vi "stim config to csv (top level vi).vi"() -> ()   [LabVIEW 2021]
uses:
  type-defs/stimulation configuration array (type def).ctl
  type-defs/stimulator configuration line cluster (type def).ctl
  type-defs/port-odor with color cluster (type def).ctl
  type-defs/port-odor ring (type def).ctl
  type-defs/odor color (type def).ctl
  type-defs/odor and manifold config cluster (type def).ctl
  type-defs/manifold configuration cluster array (type def).ctl
  type-defs/manifold configuration cluster (type def).ctl
  type-defs/manifold selection.ctl
  type-defs/single port single odor cluster.ctl
  type-defs/port number (type def).ctl
  type-defs/odor selection (type def).ctl
  type-defs/odor description array (type def).ctl
  type-defs/odor info cluster (type def).ctl
panel:
  out "csv lines out":string[](array[string])
  in  "utilized odor manifold config (none)":T1
  in  "interactive? (T)":bool=TRUE
  out "error out":errorcluster
  in  "error in (no error)":errorcluster
  in  "stim. config array in (none)":T11 {"right odor"."port-odor ring" items=["off"]; "middle odor"."port-odor ring" items=["off"]; "left odor"."port-odor ring" items=["off"]}
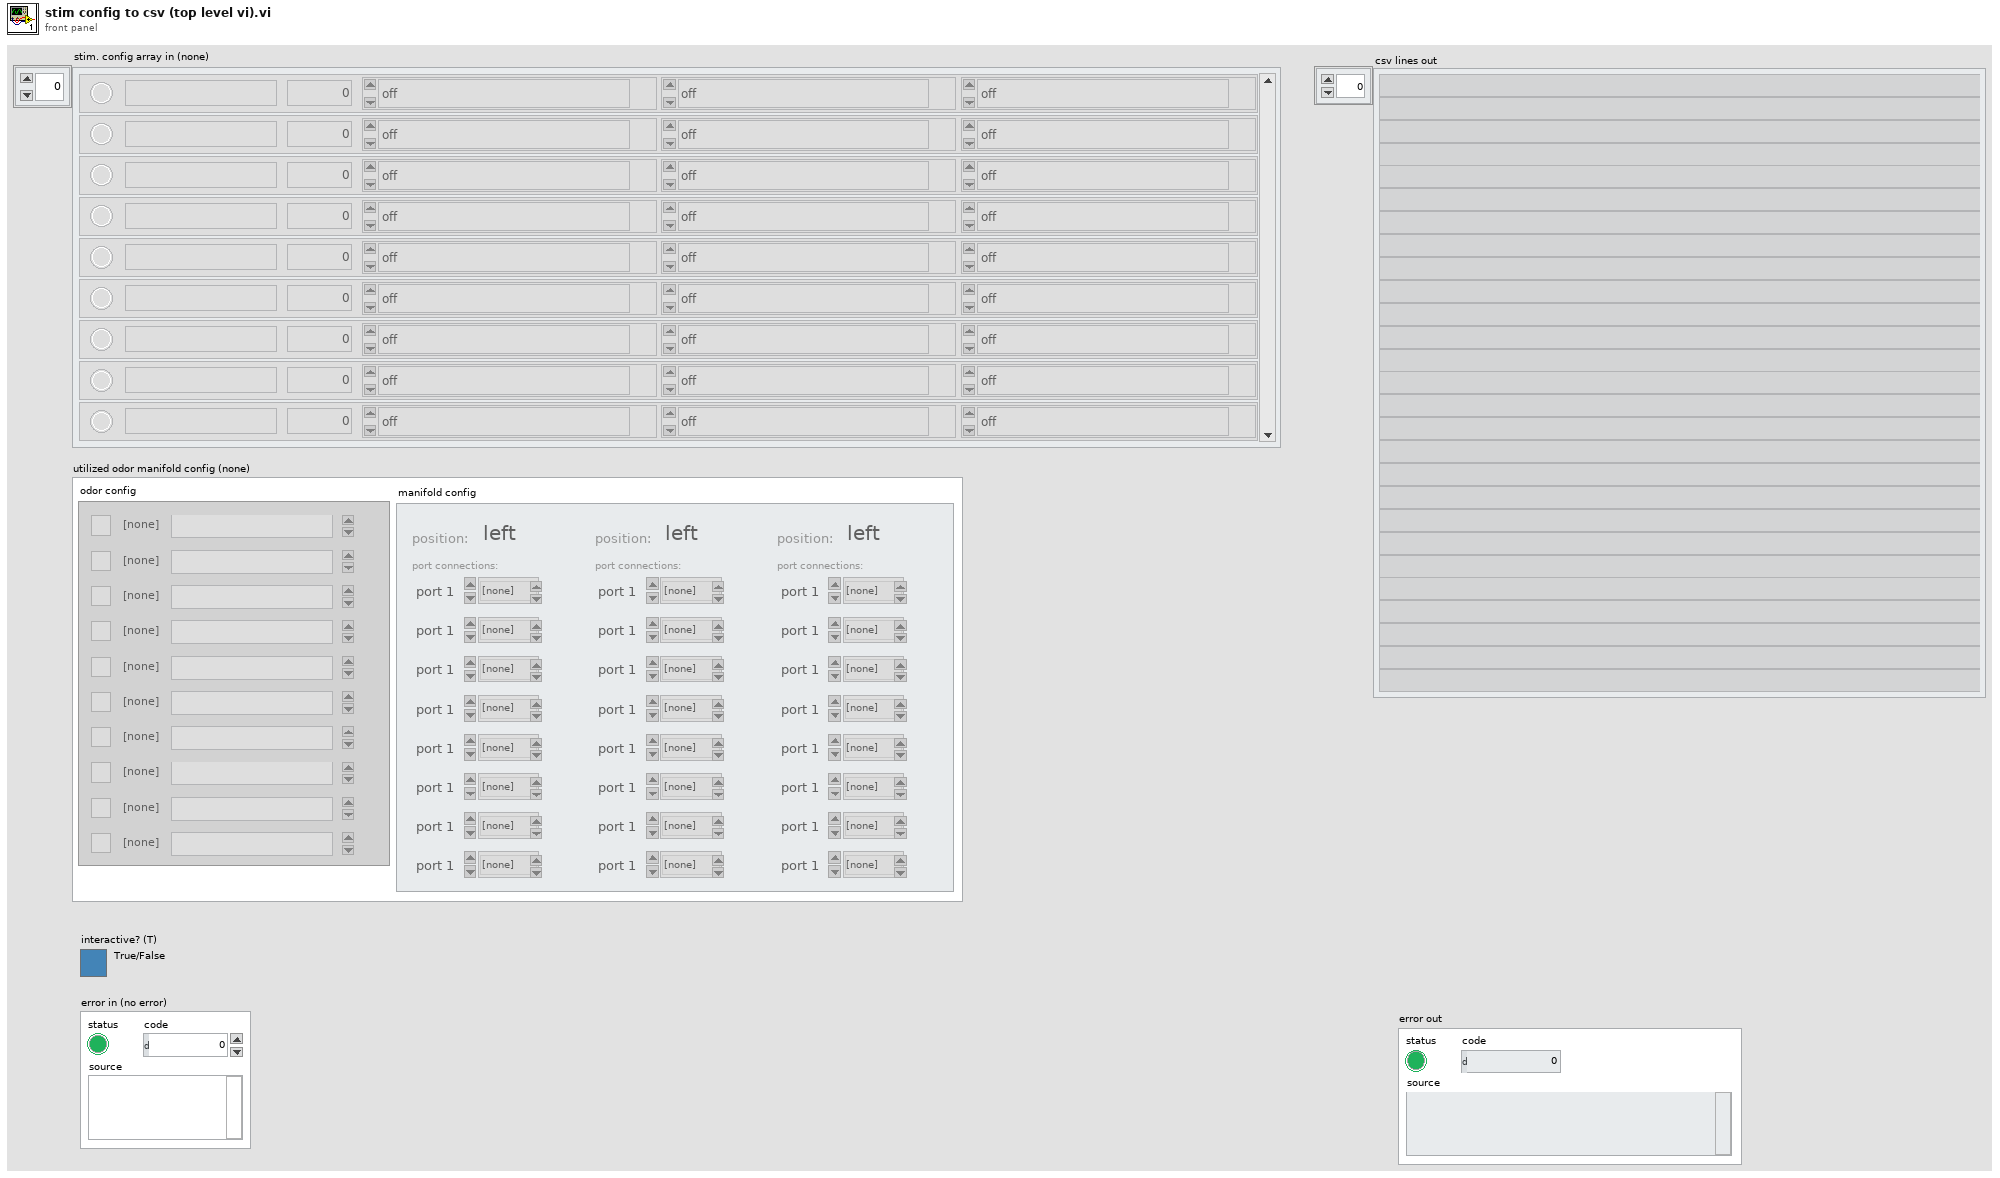
[diagram p1: front panel]
types:
  T1 = typedef "odor and manifold config cluster (type def).ctl" = cluster{"manifold config":T2, "odor config":T9}
  T2 = typedef "manifold configuration cluster array (type def).ctl" = T3[]
  T3 = typedef "manifold configuration cluster (type def).ctl" = cluster{"position:":T4, "port connections:":T5[]}
  T4 = typedef "manifold selection.ctl" = enum16{"left", "middle", "right"}
  T5 = typedef "single port single odor cluster.ctl" = cluster{"port number":T6, "connected odor":T7, "error":bool, "odor color":T8}
  T6 = typedef "port number (type def).ctl" = enum16{"port 1", "port 2", "port 3", "port 4", "port 5", "port 6", "port 7", "port 8"}
  T7 = typedef "odor selection (type def).ctl" = enum16{"[none]", "odor 1", "odor 2", "odor 3", "odor 4", "odor 5", "odor 6", "odor 7", "odor 8", "odor 9", "odor 10"}
  T8 = typedef "odor color (type def).ctl" = u16
  T9 = typedef "odor description array (type def).ctl" = T10[]
  T10 = typedef "odor info cluster (type def).ctl" = cluster{"odor channel":T7, "odor description":string, "odor color":T8, "odor channel active":bool}
  T11 = typedef "stimulation configuration array (type def).ctl" = T12[]
  T12 = typedef "stimulator configuration line cluster (type def).ctl" = cluster{"description":string, "duration, s":dbl, "left odor":T13, "middle odor":T13, "right odor":T13, "selected?":bool}
  T13 = typedef "port-odor with color cluster (type def).ctl" = cluster{"port-odor ring":T14, "odor color":T8}
  T14 = typedef "port-odor ring (type def).ctl" = u16
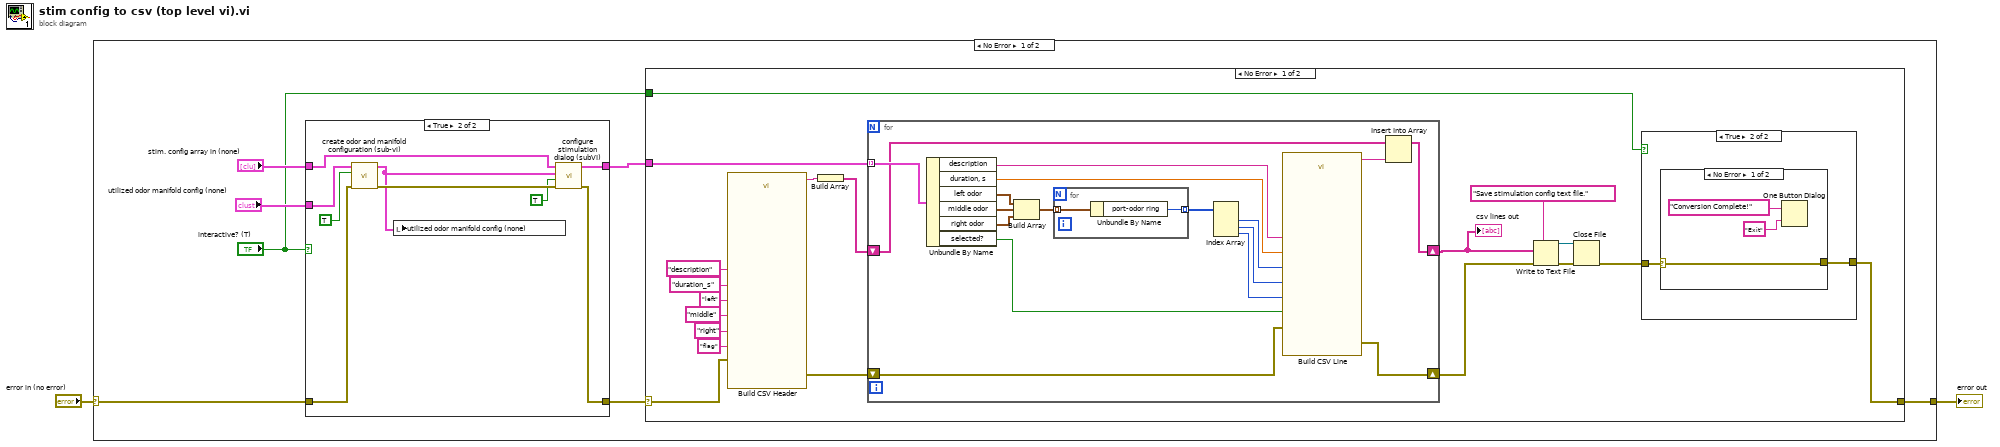
[diagram p0: block diagram]
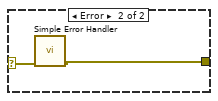
[diagram p3: hidden frame]
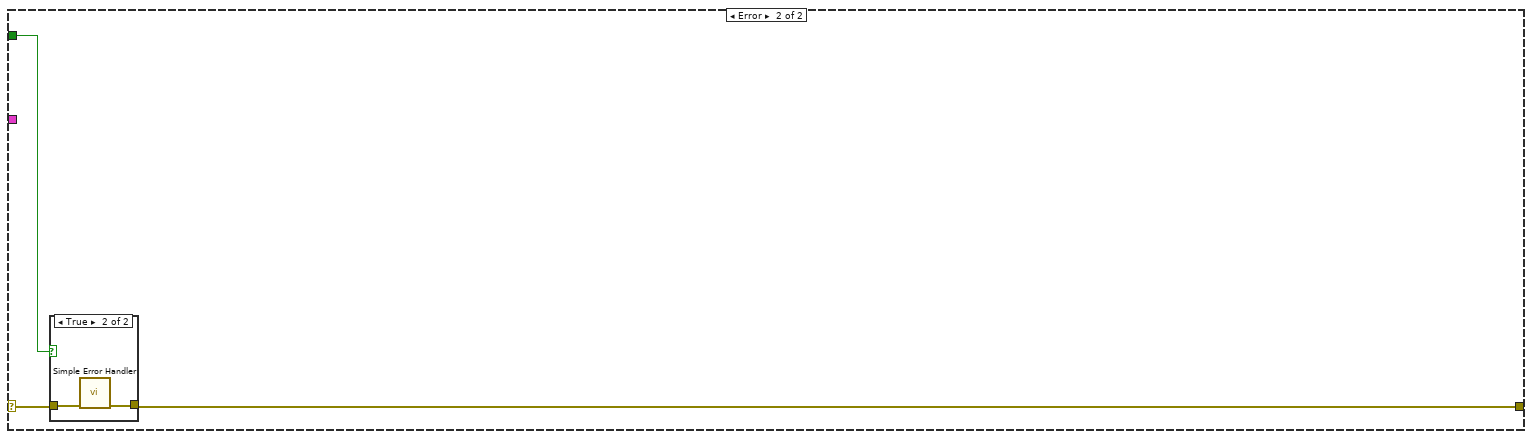
[diagram p4: hidden frame]
diagram:
  n1 = case shown="No Error" "error in (no error)" {
    selector: "error in (no error)" -> [w7 w73]
    tunnel: [w3 w73] -> w1
    frame No Error {
      n2 = case shown="True" "interactive? (T)" {
        tunnel: "stim. config array in (none)" -> [w63 w67]
        tunnel: "utilized odor manifold config (none)" -> [_ w71]
        tunnel: [w63 w70] -> w6
        tunnel: w7 -> [w62 w69]
        tunnel: [w62 w68] -> w5
        frame False {
        }
        frame True {
          n3 = call "create odor and manifold configuration (sub-vi).vi"("error in (no error)"=w69, "use initial config? (F)"=TRUE, "initial odor and manifold config (none)"=w71) -> ("error out"=w72:errorcluster, "odor and manifold config out"=w64:T1)  [unwired: 6 in, 1 out]
          n4 = local write "utilized odor manifold config (none)"(w64) -> ()
          n5 = call "configure stimulation dialog (subVI).vi"("error in (no error)"=w72, "use initial config? (F)"=TRUE, "odor and manifold config"=w64, "initial stim. config [] (empty array)"=w67) -> ("error out"=w68:errorcluster, "stim. config [] out"=w70:T11)  [unwired: 5 in, 1 out]
        }
      }
      n6 = case shown="No Error" w5 {
        selector: w5 -> [w12 w58]
        tunnel: w6 -> [w28 _]
        tunnel: "interactive? (T)" -> [w14 w56]
        tunnel: [w13 w57] -> w3
        frame No Error {
          n7 = call "Build CSV Header"("middle-stim"="middle", "flag"="flag", "description"="description", "duration_s"="duration_s", "left-stim"="left", "error in (no error)"=w12, "right-stim"="right") -> ("Result"=w21:string, "error out"=w11:errorcluster)  [unwired: 7 in]
          n8 = Build Array(w21) -> (w20:string[])
          n9 = for {
            tunnel: w28 -> [w42] mode=indexing
            shift-right: [w39] -> w15
            shift-left: w20 -> [w41]
            shift-right: [w37] -> w10
            shift-left: w11 -> [w38]
            n10 = Unbundle By Name(w42) -> ("description"=w45:string, "duration, s"=w44:dbl, "left odor"=w53:T13, "middle odor"=w52:T13, "right odor"=w51:T13, "selected?"=w43:bool)
            n11 = Build Array(w53, w52, w51) -> (w50:T13[])
            n12 = for {
              tunnel: w50 -> [w55] mode=indexing
              tunnel: [w54] -> w49 mode=indexing
              n13 = Unbundle By Name(w55) -> ("port-odor ring"=w54:T14)
            }
            n14 = Index Array(array=w49) -> (element #1=w48:T14, element #2=w47:T14, element #3=w46:T14)  [unwired: 3 in]
            n15 = call "Build CSV Line"("middle-stim"=w47, "flag"=w43, "description"=w45, "duration_s"=w44, "left-stim"=w48, "error in (no error)"=w38, "right-stim"=w46) -> ("Result"=w40:string, "error out"=w37:errorcluster)  [unwired: 7 in]
            n16 = Insert Into Array(array=w41, new element=w40) -> (w39:string[])  [unwired: 1 in]
          }
          "csv lines out" <- w15
          n17 = Write to Text File(prompt (Choose or enter file path)="Save stimulation config text file." ("prompt"), text=w15, error in=w10) -> (refnum out=w17:refnum<file>, error out=w18:errorcluster)  [unwired: 1 in, 1 out]
          n18 = Close File(refnum=w17, error in=w18) -> (error out=w16:errorcluster)  [unwired: 1 out]
          n19 = case shown="True" w14 {
            tunnel: w16 -> [w29 w31]
            tunnel: [w29 w30] -> w13
            frame False {
            }
            frame True {
              n20 = case shown="No Error" w31 {
                selector: w31 -> [w32 w36]
                tunnel: [w32 w35] -> w30
                frame No Error {
                  n21 = One Button Dialog(message="Conversion Complete!", button name ("OK")="Exit") -> ()  [unwired: 1 out]
                }
                frame Error {
                  n22 = call <vilib>:"Simple Error Handler.vi"("error in (no error)"=w36) -> ("error out"=w35:errorcluster)  [unwired: 4 in, 4 out]
                }
              }
            }
          }
        }
        frame Error {
          n23 = case shown="True" w56 {
            tunnel: w58 -> [w59 w61]
            tunnel: [w59 w60] -> w57
            frame False {
            }
            frame True {
              n24 = call <vilib>:"Simple Error Handler.vi"("error in (no error)"=w61) -> ("error out"=w60:errorcluster)  [unwired: 4 in, 4 out]
            }
          }
        }
      }
    }
    frame Error {
    }
  }
  "error out" <- w1
